vi "dfd_FXP PtByPt Cascaded SOS Form I.vi"(0 "x":T1={"value"=0, "wl"=0, "iwl"=0, "Signed"=TRUE} {"value" format="%.0x"}, 1 "coef b":i64[](array[numeric]), 2 "coef a":i64[](array[numeric]), 3 "#sec":i32, 5 "filtering statistics in":T4(array[cluster]) {"statistics information"."min value" format="%.2f"; "statistics information"."max value" format="%.2f"; "Quantizer Source" items=["Coefficients a/k"=0, "Coefficients b/v"=7, "Input"=1, "Output"=2, "Multiplicand"=3, "Product"=4, "Sum"=5, "Delay"=6]}, 6 "quantizers":T5[](array[typedef]) {"source" items=["Coef a/k"=0, "Coef b/v"=7, "Input"=1, "Output"=2, "Multiplicand"=3, "Product"=4, "Sum"=5, "Delay"=6, "Gain"=8]}, 7 "xState in":i64[](array[numeric]), 9 "yState in":i64[](array[numeric])) -> (11 "yState out":i64[](array[numeric]), 13 "xState out":i64[](array[numeric]), 14 "filtered x":T1={"value"=0, "wl"=0, "iwl"=0, "Signed"=TRUE} {"value" format="%.0x"}, 19 "filtering statistics out":T4(array[cluster]) {"statistics information"."min value" format="%.2f"; "statistics information"."max value" format="%.2f"; "Quantizer Source" items=["Coefficients a/k"=0, "Coefficients b/v"=7, "Input"=1, "Output"=2, "Multiplicand"=3, "Product"=4, "Sum"=5, "Delay"=6]})   [LabVIEW 2017, in "NI_DigFilter_FXP.lvlib"]
uses:
  <vilib>/addons/Digital Filter Design/NI_DigFilter_FXP.lvlib
  <vilib>/addons/Digital Filter Design/_Objects.llb/dfd_DFXP Data Type (scaler).ctl
  <vilib>/addons/Digital Filter Design/_Objects.llb/dfd_DFXP Operation Parameter.ctl
  <vilib>/addons/Digital Filter Design/_Objects.llb/dfd_Internal Quantization Srcs.ctl
  <vilib>/addons/Digital Filter Design/_Objects.llb/DFD Quantization Sources.ctl
  <vilib>/addons/Digital Filter Design/_Objects.llb/DFD FXP Statistics Data.ctl
  <vilib>/addons/Digital Filter Design/NI_DigFilterLicensed.lvlib
panel:
  in  "state":T1={"value"=0, "wl"=0, "iwl"=0, "Signed"=TRUE} {"value" format="%.0x"}
  in  "coef_b":T1={"value"=0, "wl"=0, "iwl"=0, "Signed"=TRUE} {"value" format="%.0x"}
  in  "coef_a":T1={"value"=0, "wl"=0, "iwl"=0, "Signed"=TRUE} {"value" format="%.0x"}
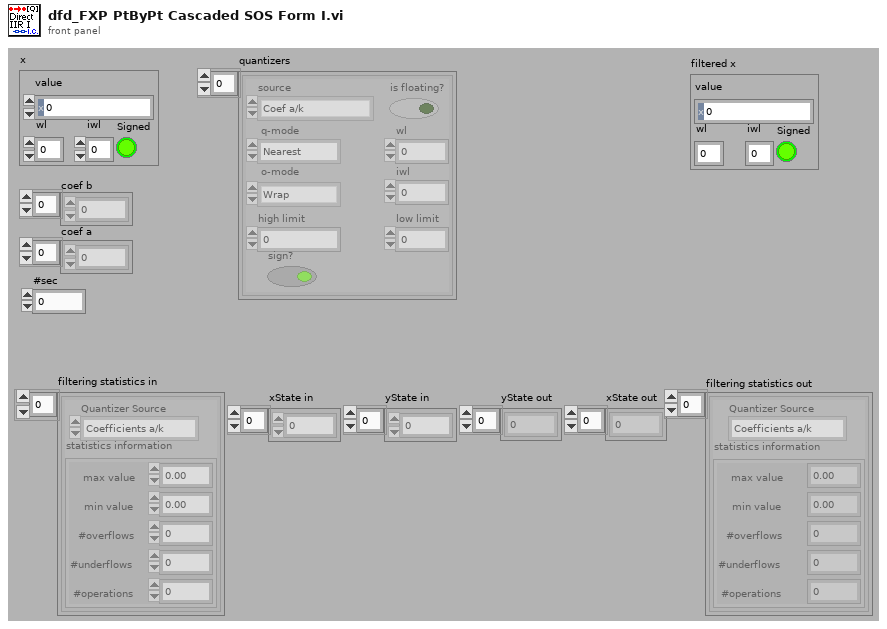
[diagram p1: front panel]
types:
  T1 = typedef "dfd_DFXP Data Type (scaler).ctl" = cluster{"value":i64, "wl":i16, "iwl":i16, "Signed":bool}
  T2 = typedef "NI_DigFilterLicensed.lvlib/DFD Quantization Sources.ctl" = u16
  T3 = typedef "NI_DigFilterLicensed.lvlib/DFD FXP Statistics Data.ctl" = cluster{"max value":ext, "min value":ext, "#overflows":i32, "#underflows":i32, "#operations":i32}
  T4 = cluster{"Quantizer Source":T2, "statistics information":T3}[]
  T5 = typedef "dfd_DFXP Operation Parameter.ctl" = cluster{"source":T6, "is floating?":bool, "o-mode":enum16{"Saturation", "Wrap"}, "q-mode":enum16{"Nearest", "Truncation"}, "wl":i16, "high limit":i64, "low limit":i64, "iwl":i16, "sign?":bool}
  T6 = typedef "NI_DigFilterLicensed.lvlib/dfd_Internal Quantization Srcs.ctl" = u16
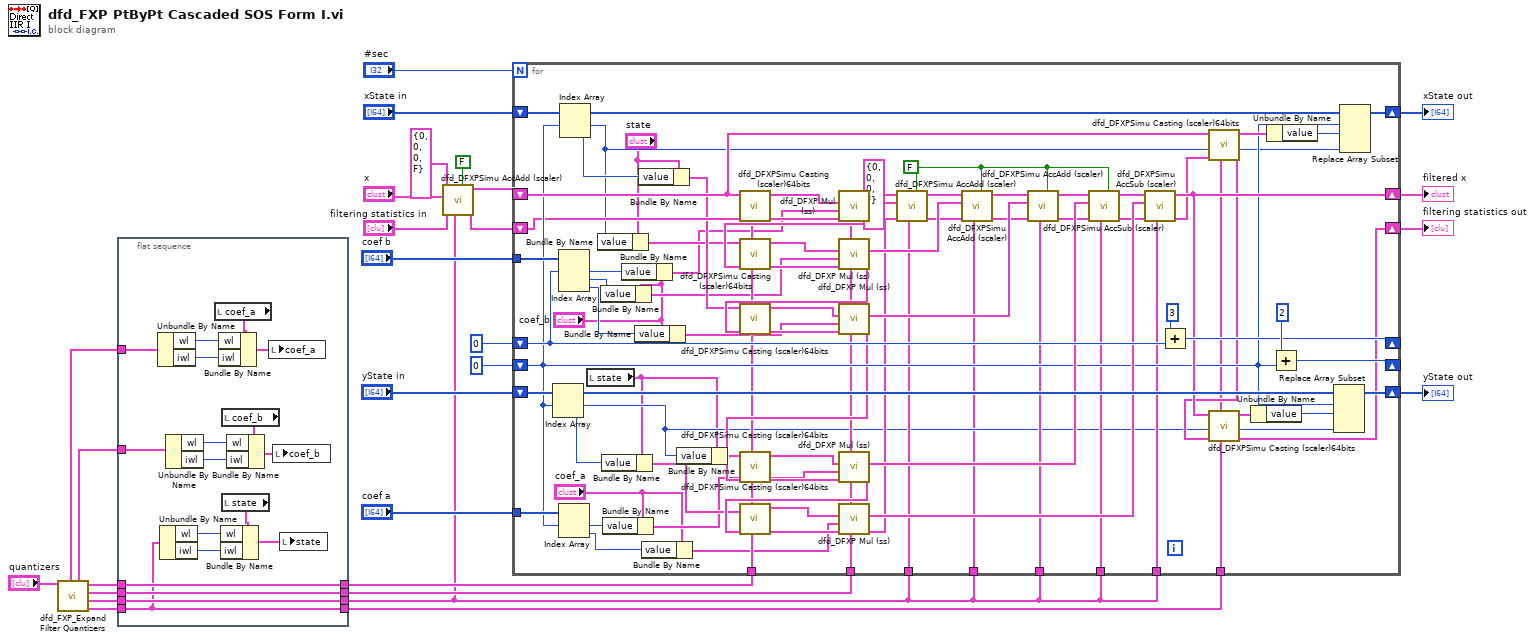
[diagram p0: block diagram]
diagram:
  n1 = call <vilib>:"dfd_FXP_Expand Filter Quantizers.vi"("FXPOPs"="quantizers") -> ("Delay"=w7:T5, "Sum"=w8:T5, "Product"=w9:T5, "Multiplicand"=w10:T5, "Coefficient b/v"=w3:T5, "Coefficient a/k"=w2:T5)  [unwired: 5 out]
  n2 = flat-sequence {
    tunnel: w7 -> [w39]
    tunnel: w10 -> [w42]
    tunnel: [w42] -> w6
    tunnel: [w41] -> w5
    tunnel: w9 -> [w41]
    tunnel: w8 -> [w40]
    tunnel: [w40] -> w1
    tunnel: [w39] -> w4
    tunnel: w3 -> [w37]
    tunnel: w2 -> [w31]
    frame #0 {
      n3 = Unbundle By Name(w31) -> ("wl"=w33:i16, "iwl"=w32:i16)
      n4 = Unbundle By Name(w39) -> ("wl"=w45:i16, "iwl"=w44:i16)
      n5 = Unbundle By Name(w37) -> ("wl"=w34:i16, "iwl"=w38:i16)
      n6 = local read "coef_a"() -> (w29:T1)
      n7 = Bundle By Name(cluster=w29, "wl"=w33, "iwl"=w32) -> (w30:T1)
      n8 = local read "coef_b"() -> (w35:T1)
      n9 = local read "state"() -> (w46:T1)
      n10 = Bundle By Name(cluster=w46, "wl"=w45, "iwl"=w44) -> (w43:T1)
      n11 = Bundle By Name(cluster=w35, "wl"=w34, "iwl"=w38) -> (w36:T1)
      n12 = local write "coef_a"(w30) -> ()
      n13 = local write "coef_b"(w36) -> ()
      n14 = local write "state"(w43) -> ()
    }
  }
  n15 = call <vilib>:"dfd_DFXPSimu AccAdd (scaler).vi"("quantize output? (T)"=FALSE ("quantize output?"), "op params"=w1, "filtering statistics in"="filtering statistics in", "addend"="x", "acc in"=T1 {"value"=0, "wl"=0, "iwl"=0, "Signed"=FALSE}) -> ("filtering statistics out"=w13:T4, "acc out"=w15:T1)  [unwired: 5 out]
  n16 = for {
    N: "#sec" -> [_]
    shift-right: [w125] -> w25
    shift-left: "yState in" -> [w126]
    shift-right: [w127] -> w27
    shift-left: "xState in" -> [w128]
    shift-right: [w124] -> _
    shift-left: 0 -> [w104]
    shift-right: [w112] -> w19
    shift-left: w15 -> [w106]
    shift-right: [w121] -> _
    shift-left: 0 -> [w119]
    tunnel: "coef b" -> [w120]
    tunnel: "coef a" -> [w118]
    tunnel: w6 -> [w87]
    tunnel: w5 -> [w86]
    tunnel: w1 -> [w47]
    tunnel: w1 -> [w83]
    tunnel: w1 -> [w84]
    tunnel: w1 -> [w85]
    tunnel: w4 -> [w66]
    shift-right: [w88] -> w17
    shift-left: w13 -> [w103]
    tunnel: w1 -> [w81]
    w65 = FALSE ("quantize output?")
    n17 = Index Array(array=w126, index #1=w104) -> (element #1=w51:i64, element #2=w107:i64)  [unwired: 1 in]
    n18 = Index Array(array=w120, index #1=w119) -> (element #1=w75:i64, element #2=w73:i64, element #3=w71:i64)  [unwired: 2 in]
    n19 = Index Array(array=w118, index #1=w104) -> (element #1=w69:i64, element #2=w67:i64)  [unwired: 1 in]
    n20 = Index Array(array=w128, index #1=w104) -> (element #1=w63:i64, element #2=w105:i64)  [unwired: 1 in]
    n21 = local read "state"() -> (w49:T1)
    n22 = Bundle By Name(cluster="state", "value"=w63) -> (w62:T1)
    n23 = Bundle By Name(cluster="coef_b", "value"=w73) -> (w57:T1)
    n24 = Bundle By Name(cluster=w49, "value"=w107) -> (w55:T1)
    n25 = Bundle By Name(cluster="coef_a", "value"=w69) -> (w54:T1)
    n26 = Bundle By Name(cluster="coef_b", "value"=w75) -> (w59:T1)
    n27 = Bundle By Name(cluster="coef_b", "value"=w71) -> (w58:T1)
    n28 = Bundle By Name(cluster="state", "value"=w105) -> (w64:T1)
    n29 = Bundle By Name(cluster="coef_a", "value"=w67) -> (w53:T1)
    n30 = Bundle By Name(cluster=w49, "value"=w51) -> (w50:T1)
    n31 = call <vilib>:"dfd_DFXPSimu Casting (scaler)64bits.vi"("op params"=w87, "filtering statistics in"=w103, "Value in"=w106) -> ("filtering statistics out"=w102:T4, "Value out"=w76:T1)  [unwired: 2 in, 5 out]
    n32 = call <vilib>:"dfd_DFXP Mul (ss).vi"("op params"=w86, "filtering statistics in"=w102, "Value in 2"=w59, "Value in"=w76) -> ("filtering statistics out"=w101:T4, "Value out"=w78:T1)  [unwired: 6 out]
    n33 = call <vilib>:"dfd_DFXPSimu Casting (scaler)64bits.vi"("op params"=w87, "filtering statistics in"=w101, "Value in"=w62) -> ("filtering statistics out"=w100:T4, "Value out"=w74:T1)  [unwired: 2 in, 5 out]
    n34 = call <vilib>:"dfd_DFXP Mul (ss).vi"("op params"=w86, "filtering statistics in"=w100, "Value in 2"=w57, "Value in"=w74) -> ("filtering statistics out"=w99:T4, "Value out"=w117:T1)  [unwired: 6 out]
    n35 = call <vilib>:"dfd_DFXPSimu Casting (scaler)64bits.vi"("op params"=w87, "filtering statistics in"=w99, "Value in"=w64) -> ("filtering statistics out"=w98:T4, "Value out"=w72:T1)  [unwired: 2 in, 5 out]
    n36 = call <vilib>:"dfd_DFXP Mul (ss).vi"("op params"=w86, "filtering statistics in"=w98, "Value in 2"=w58, "Value in"=w72) -> ("filtering statistics out"=w97:T4, "Value out"=w115:T1)  [unwired: 6 out]
    n37 = call <vilib>:"dfd_DFXPSimu Casting (scaler)64bits.vi"("op params"=w87, "filtering statistics in"=w97, "Value in"=w50) -> ("filtering statistics out"=w96:T4, "Value out"=w70:T1)  [unwired: 2 in, 5 out]
    n38 = call <vilib>:"dfd_DFXP Mul (ss).vi"("op params"=w86, "filtering statistics in"=w96, "Value in 2"=w54, "Value in"=w70) -> ("filtering statistics out"=w95:T4, "Value out"=w109:T1)  [unwired: 6 out]
    n39 = call <vilib>:"dfd_DFXPSimu Casting (scaler)64bits.vi"("op params"=w87, "filtering statistics in"=w95, "Value in"=w55) -> ("filtering statistics out"=w94:T4, "Value out"=w68:T1)  [unwired: 2 in, 5 out]
    n40 = call <vilib>:"dfd_DFXP Mul (ss).vi"("op params"=w86, "filtering statistics in"=w94, "Value in 2"=w53, "Value in"=w68) -> ("filtering statistics out"=w80:T4, "Value out"=w108:T1)  [unwired: 6 out]
    n41 = call <vilib>:"dfd_DFXPSimu AccAdd (scaler).vi"("quantize output? (T)"=w65, "op params"=w81, "filtering statistics in"=w80, "addend"=w78, "acc in"=T1 {"value"=0, "wl"=0, "iwl"=0, "Signed"=FALSE}) -> ("filtering statistics out"=w79:T4, "acc out"=w82:T1)  [unwired: 5 out]
    n42 = call <vilib>:"dfd_DFXPSimu AccAdd (scaler).vi"("quantize output? (T)"=w65, "op params"=w47, "filtering statistics in"=w79, "addend"=w117, "acc in"=w82) -> ("filtering statistics out"=w93:T4, "acc out"=w116:T1)  [unwired: 5 out]
    n43 = call <vilib>:"dfd_DFXPSimu AccAdd (scaler).vi"("quantize output? (T)"=w65, "op params"=w83, "filtering statistics in"=w93, "addend"=w115, "acc in"=w116) -> ("filtering statistics out"=w92:T4, "acc out"=w114:T1)  [unwired: 5 out]
    n44 = call <vilib>:"dfd_DFXPSimu AccSub (scaler).vi"("quantize output?(T)"=w65, "op params"=w84, "filtering statistics in"=w92, "addend"=w109, "acc in"=w114) -> ("filtering statistics out"=w91:T4, "acc out"=w113:T1)  [unwired: 5 out]
    n45 = call <vilib>:"dfd_DFXPSimu AccSub (scaler).vi"("op params"=w85, "filtering statistics in"=w91, "addend"=w108, "acc in"=w113) -> ("filtering statistics out"=w90:T4, "acc out"=w112:T1)  [unwired: 1 in, 5 out]
    n46 = Add(x=3, y=w119) -> (x+y=w121:i32)
    n47 = call <vilib>:"dfd_DFXPSimu Casting (scaler)64bits.vi"("op params"=w66, "filtering statistics in"=w90, "Value in"=w106) -> ("filtering statistics out"=w89:T4, "Value out"=w110:T1)  [unwired: 1 in, 6 out]
    n48 = call <vilib>:"dfd_DFXPSimu Casting (scaler)64bits.vi"("op params"=w66, "filtering statistics in"=w89, "Value in"=w112) -> ("filtering statistics out"=w88:T4, "Value out"=w111:T1)  [unwired: 1 in, 6 out]
    n49 = Unbundle By Name(w111) -> ("value"=w48:i64)
    n50 = Unbundle By Name(w110) -> ("value"=w60:i64)
    n51 = Add(x=2 ("y"), y=w104) -> (x+y=w124:i32)
    n52 = Replace Array Subset(array=w126, new element #1=w48, index #1=w104, new element #2=w51) -> (w125:i64[])  [unwired: 1 in]
    n53 = Replace Array Subset(array=w128, new element #1=w60, index #1=w104, new element #2=w63) -> (w127:i64[])  [unwired: 1 in]
  }
  "filtered x" <- w19
  "xState out" <- w27
  "yState out" <- w25
  "filtering statistics out" <- w17
